vi "同步局域网时间.vi"() -> ()   [LabVIEW 2014]
panel:
  in  "stop":bool
  in  "时间同步":bool
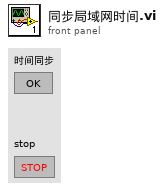
[diagram p1: front panel]
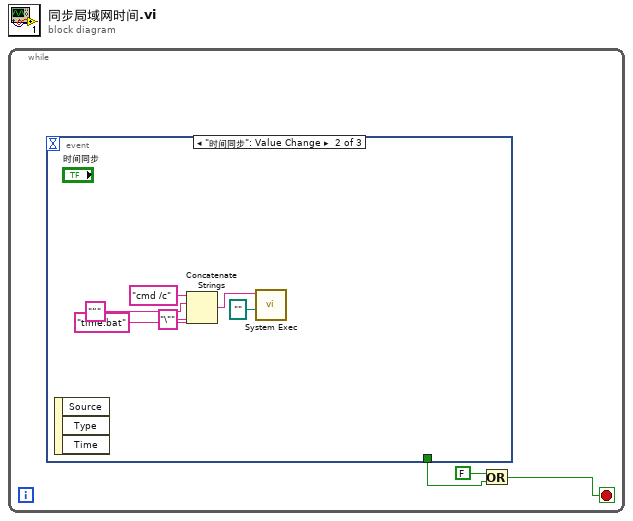
[diagram p0: block diagram]
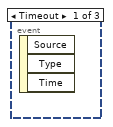
[diagram p2: hidden frame]
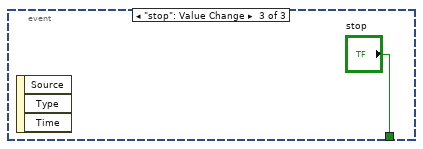
[diagram p3: hidden frame]
diagram:
  n1 = while {
    stop <- w1 stop-if-true
    n2 = event shown="[1] \"时间同步\": Value Change" {
      selector: _ -> [_ _ _]
      dyn-events: _ -> [_ _ _]
      timeout: _ -> [_ _ _]
      tunnel: [_ _ "stop"] -> w2
      event Timeout {
        n3 = event-data() -> ()  [unwired: 1 in, 3 out]
      }
      event "时间同步": Value Change {
        n4 = event-data() -> ()  [unwired: 1 in, 3 out]
        n5 = Concatenate Strings("cmd /c" ("string"), "“" ("string"), "time.bat" ("string"), "\"" ("string")) -> (w9:string)
        n6 = call <vilib>:"System Exec.vi"("working directory"=path "", "command line"=w9) -> ()  [unwired: 6 in, 4 out]
      }
      event "stop": Value Change {
        n7 = event-data() -> ()  [unwired: 1 in, 3 out]
      }
    }
    n8 = Or(x=FALSE, y=w2) -> (x .or. y?=w1:bool)
  }
